vi "Run VI Method With Arguments.vi"() -> ()   [LabVIEW 2020]
panel:
  in  "delayInSeconds":dbl
  in  "stop":bool
  out "iterations":i32
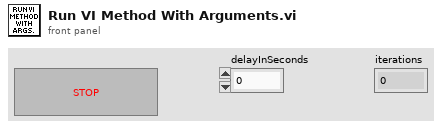
[diagram p1: front panel]
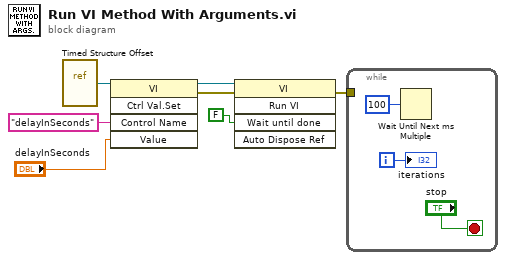
[diagram p0: block diagram]
diagram:
  n1 = vi-ref "Timed Structure Offset.vi"() -> (w7:refnum<vi>)
  n2 = invoke class="VI" method="Ctrl Val.Set"(reference=w7, "Control Name"="delayInSeconds", "Value"="delayInSeconds") -> (reference out=w6:refnum<vi>, error out=w1:errorcluster)  [unwired: 2 in, 3 out]
  n3 = invoke class="VI" method="Run VI"(reference=w6, error in=w1, "Wait until done"=FALSE ("Wait Until Done")) -> (error out=w2:errorcluster)  [unwired: 2 in, 4 out]
  n4 = while {
    tunnel: w2 -> [_]
    i -> [w10]
    stop <- "stop" stop-if-true
    n5 = Wait Until Next ms Multiple(millisecond multiple=u32 100) -> ()  [unwired: 1 out]
    "iterations" <- w10
  }
